vi "display image.vi"(3 "error in":errorcluster, 5 "Camera Handle In":u32, 6 "Image Handle":u32) -> (0 "error out":errorcluster, 1 "Camera Handle Out":u32, 2 "Data Handle":u32, 4 "Image array":u8[][](array[numeric]) caption="Array uint 16")   [LabVIEW 2012]
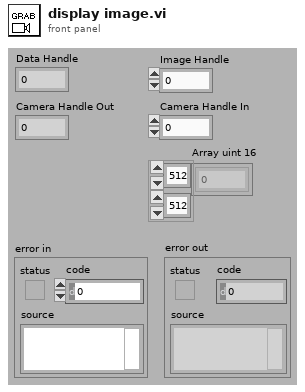
[diagram p1: front panel]
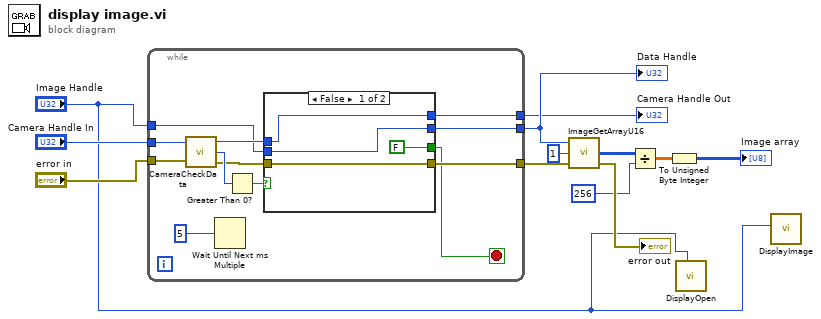
[diagram p0: block diagram]
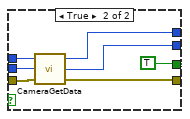
[diagram p2: hidden frame]
diagram:
  n1 = while {
    tunnel: "error in" -> [w20]
    tunnel: [w19] -> w10
    tunnel: "Image Handle" -> [w18]
    tunnel: "Camera Handle In" -> [w17]
    tunnel: [w15] -> w12
    tunnel: [w14] -> w9
    stop <- w13 stop-if-true
    n2 = call <userlib>:"CameraCheckData.vi"("Camera Handle"=w17, "error in"=w20) -> ("Camera Handle"=w23:u32, "Number Of Frames Available"=w22:i32, "error out"=w21:errorcluster)
    n3 = Wait Until Next ms Multiple(millisecond multiple=5) -> ()  [unwired: 1 out]
    n4 = Greater Than 0?(x=w22) -> (x > 0?=w24:bool)
    n5 = case shown="False" w24 {
      tunnel: w23 -> [w25 w35]
      tunnel: w21 -> [w28 w34]
      tunnel: [w28 w31] -> w19
      tunnel: [FALSE TRUE] -> w13
      tunnel: w18 -> [w26 w32]
      tunnel: [w26 w30] -> w15
      tunnel: [w25 w29] -> w14
      frame False {
      }
      frame True {
        n6 = call <userlib>:"CameraGetData.vi"("error in"=w34, "Data Handle"=w32, "Camera Handle"=w35) -> ("error out"=w31:errorcluster, "Data Handle"=w30:u32, "Camera Handle"=w29:u32)
      }
    }
  }
  "Data Handle" <- w12
  "Camera Handle Out" <- w9
  n7 = call <userlib>:"ImageGetArrayU16.vi"("error in"=w10, "Z position"=u32 1, "Image Handle"=w12) -> ("error out"=→"error out":errorcluster, "Array uint 16"=w5:u16[][])  [unwired: 1 out]
  n8 = Divide(x=w5, y=u32 256 ("Z position")) -> (x/y=w1:dbl[][])
  n9 = To Unsigned Byte Integer(number=w1) -> (unsigned 8bit integer=→"Image array":u8[][])
  n10 = call <userlib>:"DisplayOpen.vi"("Image Handle"="Image Handle") -> ()  [unwired: 5 in, 2 out]
  n11 = call <userlib>:"DisplayImage.vi"("Image Handle"="Image Handle") -> ()  [unwired: 3 in, 2 out]
